vi "Get sr850 Formated Parameters VISA.VI"(8 "error in (no error)":errorcluster, 10 "Initial String":string, 11 "VISA resource name":refnum<visa-resource-name>) -> (0 "error out":errorcluster, 1 "Time Constant":dbl format="%.2e", 2 "Sensitivity":dbl format="%.4e", 3 "Frequency":dbl format="%.2e", 4 "Phase":dbl format="%.2f", 5 "Oscillator voltage":dbl format="%.2e", 6 "Parameters":string="SR850 Lockin Settings", 7 "Filter Slope":i32)   [LabVIEW 2015]
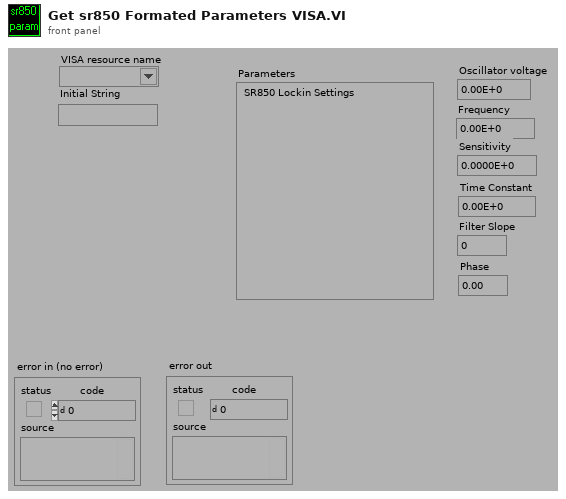
[diagram p1: front panel]
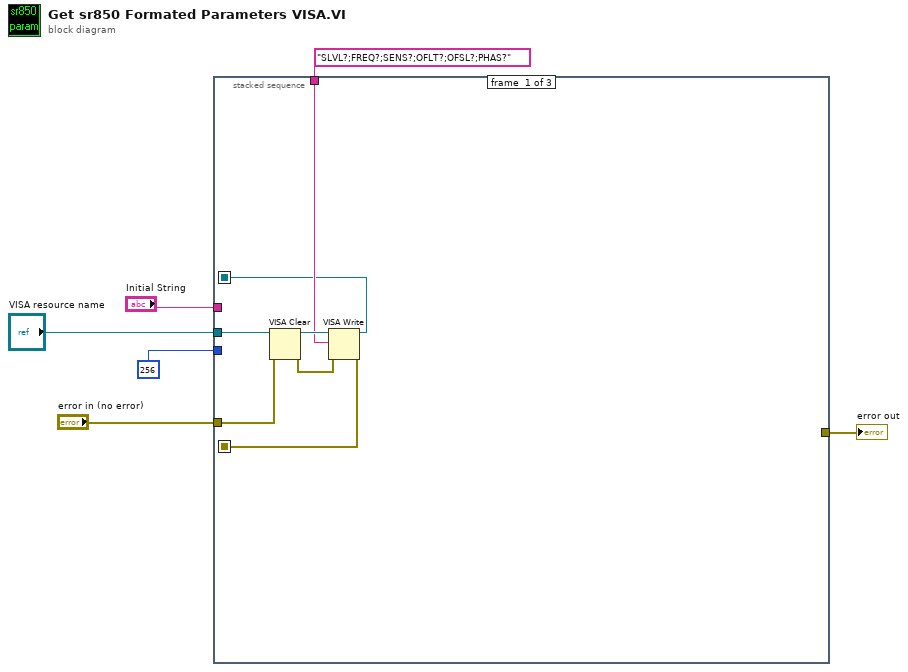
[diagram p0: block diagram]
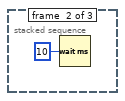
[diagram p2: hidden frame]
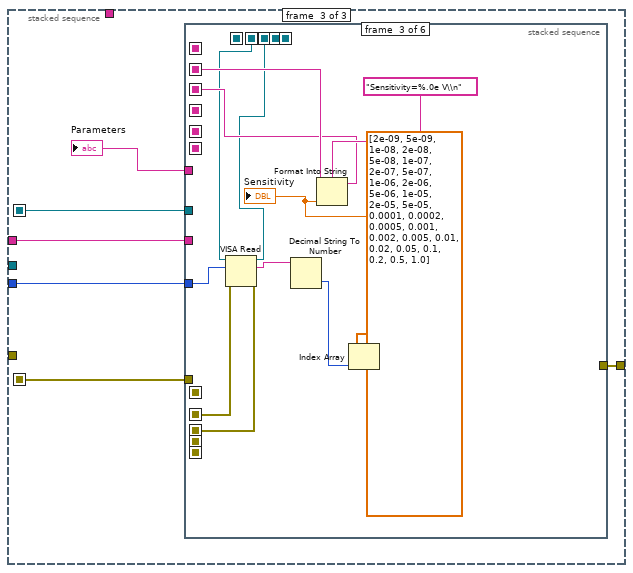
[diagram p3: hidden frame]
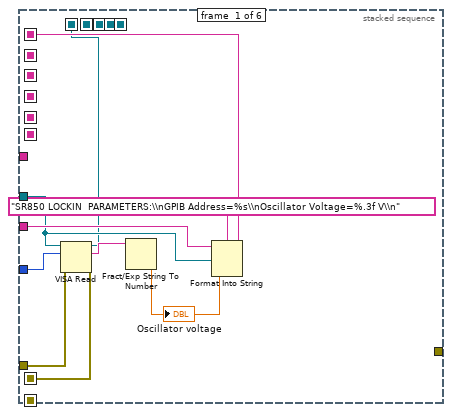
[diagram p4: hidden frame]
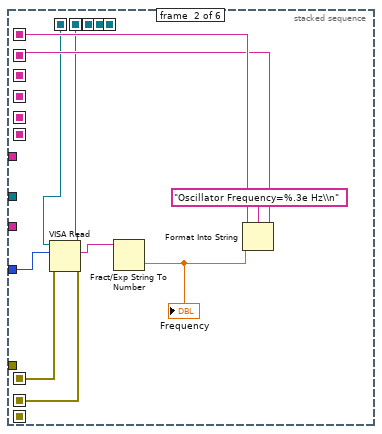
[diagram p5: hidden frame]
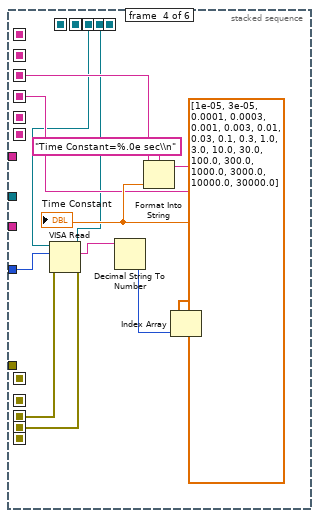
[diagram p6: hidden frame]
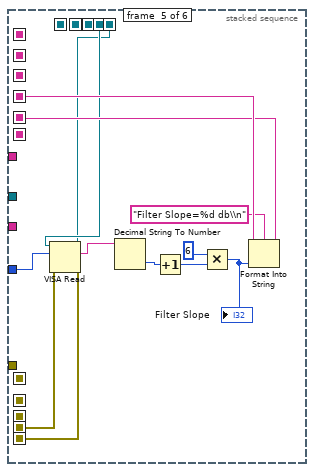
[diagram p7: hidden frame]
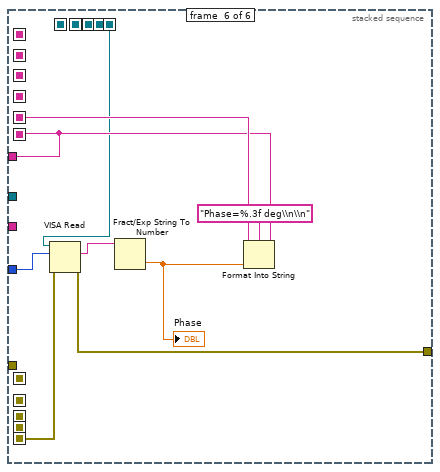
[diagram p8: hidden frame]
diagram:
  n1 = stacked-sequence {
    seq-local: [w11 _ _] -> [_ _ w17]
    seq-local: [w7 _ _] -> [_ _ w15]
    tunnel: "VISA resource name" -> [w10 _ _]
    tunnel: u32 256 ("count") -> [_ _ w20]
    tunnel: "SLVL?;FREQ?;SENS?;OFLT?;OFSL?;PHAS?" ("data string") -> [w8 _ _]
    tunnel: "Initial String" -> [_ _ w18]
    tunnel: "error in (no error)" -> [w13 _ _]
    tunnel: [_ _ w16] -> w2
    frame #0 {
      n2 = VISA Clear(VISA resource name=w10, error in (no error)=w13) -> (VISA resource name out=w9:refnum<visa-resource-name>, error out=w12:errorcluster)
      n3 = VISA Write(VISA resource name=w9, write buffer=w8, error in (no error)=w12) -> (VISA resource name out=w7:refnum<visa-resource-name>, error out=w11:errorcluster)  [unwired: 1 out]
    }
    frame #1 {
      n4 = Wait (ms)(milliseconds to wait=u32 10) -> ()  [unwired: 1 out]
    }
    frame #2 {
      n5 = stacked-sequence {
        seq-local: [w28 _ _ _ _ _] -> [_ w38 _ _ _ _]
        seq-local: [_ w37 _ _ _ _] -> [_ _ w47 _ _ _]
        seq-local: [_ _ w46 _ _ _] -> [_ _ _ w59 _ _]
        seq-local: [_ _ _ w58 _ _] -> [_ _ _ _ w72 _]
        seq-local: [_ _ _ _ w71 _] -> [_ _ _ _ _ w83]
        seq-local: [_ _ _ _ _ w82] -> [_ _ _ _ _ _]
        seq-local: [w25 _ _ _ _ _] -> [_ w35 _ _ _ _]
        seq-local: [_ w34 _ _ _ _] -> [_ _ w45 _ _ _]
        seq-local: [_ _ w44 _ _ _] -> [_ _ _ w57 _ _]
        seq-local: [_ _ _ w56 _ _] -> [_ _ _ _ w69 _]
        seq-local: [_ _ _ _ w68 _] -> [_ _ _ _ _ w81]
        seq-local: [w21 _ _ _ _ _] -> [_ w32 _ _ _ _]
        seq-local: [_ w31 _ _ _ _] -> [_ _ w43 _ _ _]
        seq-local: [_ _ w41 _ _ _] -> [_ _ _ w55 _ _]
        seq-local: [_ _ _ w53 _ _] -> [_ _ _ _ w67 _]
        seq-local: [_ _ _ _ w65 _] -> [_ _ _ _ _ w79]
        tunnel: w20 -> [w30 w36 w52 w64 w77 w86]
        tunnel: [_ _ _ _ _ w82] -> w19
        tunnel: w18 -> [w27 _ _ _ _ _]
        tunnel: w17 -> [w26 _ _ _ _ _]
        tunnel: [_ _ _ _ _ w80] -> w16
        tunnel: w15 -> [w23 _ _ _ _ _]
        frame #0 {
          n6 = VISA Read(VISA resource name=w23, byte count=w30, error in (no error)=w26) -> (VISA resource name out=w21:refnum<visa-resource-name>, read buffer=w22:string, error out=w25:errorcluster)  [unwired: 1 out]
          n7 = Fract/Exp String To Number(string=w22) -> (number=w24:dbl)  [unwired: 4 out]
          "Oscillator voltage" <- w24
          n8 = Format Into String(format string="SR850 LOCKIN  PARAMETERS:\\nGPIB Address=%s\\nOscillator Voltage=%.3f V\\n", initial string=w27, w23, w24) -> (resulting string=w28:string)  [unwired: 1 in, 1 out]
        }
        frame #1 {
          n9 = VISA Read(VISA resource name=w32, byte count=w36, error in (no error)=w35) -> (VISA resource name out=w31:refnum<visa-resource-name>, read buffer=w33:string, error out=w34:errorcluster)  [unwired: 1 out]
          n10 = Fract/Exp String To Number(string=w33) -> (number=w39:dbl)  [unwired: 4 out]
          "Frequency" <- w39
          n11 = Format Into String(format string="Oscillator Frequency=%.3e Hz\\n", initial string=w38, w39) -> (resulting string=w37:string)  [unwired: 1 in, 1 out]
        }
        frame #2 {
          n12 = VISA Read(VISA resource name=w43, byte count=w52, error in (no error)=w45) -> (VISA resource name out=w41:refnum<visa-resource-name>, read buffer=w42:string, error out=w44:errorcluster)  [unwired: 1 out]
          n13 = Decimal String To Number(string=w42) -> (number=w50:i32)  [unwired: 3 out]
          n14 = Index Array(array=dbl[] [2e-09, 5e-09, 1e-08, 2e-08, 5e-08, 1e-07, 2e-07, 5e-07, 1e-06, 2e-06, 5e-06, 1e-05, 2e-05, 5e-05, 0.0001, 0.0002, 0.0005, 0.001, 0.002, 0.005, 0.01, 0.02, 0.05, 0.1, 0.2, 0.5, 1.0], index=w50) -> (element=w49:dbl)
          "Sensitivity" <- w49
          n15 = Format Into String(format string="Sensitivity=%.0e V\\n", initial string=w47, w49) -> (resulting string=w46:string)  [unwired: 1 in, 1 out]
        }
        frame #3 {
          n16 = VISA Read(VISA resource name=w55, byte count=w64, error in (no error)=w57) -> (VISA resource name out=w53:refnum<visa-resource-name>, read buffer=w54:string, error out=w56:errorcluster)  [unwired: 1 out]
          n17 = Decimal String To Number(string=w54) -> (number=w63:i32)  [unwired: 3 out]
          n18 = Index Array(array=dbl[] [1e-05, 3e-05, 0.0001, 0.0003, 0.001, 0.003, 0.01, 0.03, 0.1, 0.3, 1.0, 3.0, 10.0, 30.0, 100.0, 300.0, 1000.0, 3000.0, 10000.0, 30000.0], index=w63) -> (element=w60:dbl)
          "Time Constant" <- w60
          n19 = Format Into String(format string="Time Constant=%.0e sec\\n", initial string=w59, w60) -> (resulting string=w58:string)  [unwired: 1 in, 1 out]
        }
        frame #4 {
          n20 = VISA Read(VISA resource name=w67, byte count=w77, error in (no error)=w69) -> (VISA resource name out=w65:refnum<visa-resource-name>, read buffer=w66:string, error out=w68:errorcluster)  [unwired: 1 out]
          n21 = Decimal String To Number(string=w66) -> (number=w76:i32)  [unwired: 3 out]
          n22 = Increment(x=w76) -> (x+1=w74:i32)
          n23 = Multiply(x=6, y=w74) -> (x*y=w73:i32)
          "Filter Slope" <- w73
          n24 = Format Into String(format string="Filter Slope=%d db\\n", initial string=w72, w73) -> (resulting string=w71:string)  [unwired: 1 in, 1 out]
        }
        frame #5 {
          n25 = VISA Read(VISA resource name=w79, byte count=w86, error in (no error)=w81) -> (read buffer=w78:string, error out=w80:errorcluster)  [unwired: 2 out]
          n26 = Fract/Exp String To Number(string=w78) -> (number=w85:dbl)  [unwired: 4 out]
          "Phase" <- w85
          n27 = Format Into String(format string="Phase=%.3f deg\\n\\n", initial string=w83, w85) -> (resulting string=w82:string)  [unwired: 1 in, 1 out]
        }
      }
      "Parameters" <- w19
    }
  }
  "error out" <- w2
